vi "CheckPlotVisability.vi"(10 "Array":cluster{"x0":dbl, "df":dbl, dbl[]}[](array[cluster]), 11 "WaveformGraph in":refnum<vi>) -> (1 "rescale":bool, 3 "WaveformGraph out":refnum<vi>)   [LabVIEW 2022 SP3]
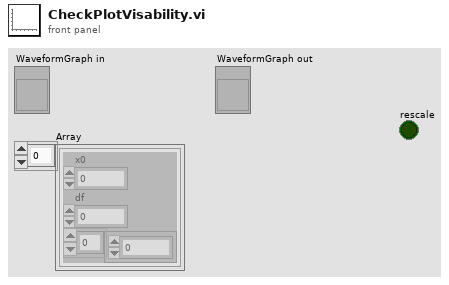
[diagram p1: front panel]
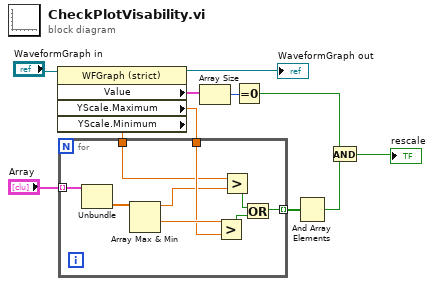
[diagram p0: block diagram]
diagram:
  n1 = property class="WFGraph (strict)"(reference="WaveformGraph in") -> (reference out=→"WaveformGraph out":refnum<vi>, "Value"=w9:cluster{dbl, "df":dbl, dbl[]}[], "YScale.Maximum"=w6:dbl, "YScale.Minimum"=w5:dbl)  [unwired: 1 in, 1 out]
  n2 = for {
    tunnel: "Array" -> [w20] mode=indexing
    tunnel: w6 -> [w17]
    tunnel: w5 -> [w15]
    tunnel: [w12] -> w4 mode=indexing
    n3 = Unbundle(w20) -> (w19:dbl[])  [unwired: 2 out]
    n4 = Array Max & Min(array=w19) -> (max value=w16:dbl, min value=w18:dbl)  [unwired: 2 out]
    n5 = Greater?(x=w18, y=w17) -> (0:w13:bool)
    n6 = Greater?(x=w15, y=w16) -> (0:w14:bool)
    n7 = Or(x=w14, y=w13) -> (x .or. y?=w12:bool)
  }
  n8 = Array Size(array=w9) -> (size(s)=w8:i32)
  n9 = Equal To 0?(x=w8) -> (x = 0?=w3:bool)
  n10 = And Array Elements(Boolean array=w4) -> (logical AND=w2:bool)
  n11 = And(x=w3, y=w2) -> (x .and. y?=→"rescale":bool)
